vi "main.vi"() -> ()   [LabVIEW 2025]
uses:
  3a10f0c5-8fb2-42eb-acf3-e30270466858.vi
  global/HP amount.vi
  global/bullet amount.vi
  global/difficulty.vi
  global/item amount.vi
  global/demo mode.vi
panel:
  out "Array":bool[](array[boolean])
  out "Player did stuff":bool
  out "Guess bullet type":i32
  out "Numeric":u32
  in  "item array 2":u32[](array[numeric])
  in  "item array":u32[](array[numeric])
  out "item picture 2":u32[](array[ring])
  out "button 2":bool[](array[boolean])
  in  "button":bool[](array[boolean])
  out "item picture":u32[](array[ring])
  out "String":string
  out "chamber ind":u32[](array[ring])
  out "End of action":bool
  out "Total HP var":u32
  out "P1's turn":bool
  out "Chamber":i32[](array[numeric])
  in  "Hit other":bool
  in  "Hit self":bool
  out "STOP":bool
  out "Difficulty":u32
  out "P1 HP var":i32
  out "AI HP var":i32
  out "Item amount":u32
  out "Total rounds":u32
  out "Empty rounds":u32
  out "Live rounds":u32
  out "Player HP ind":T1
  out "AI HP ind":T1
  out "round":u32
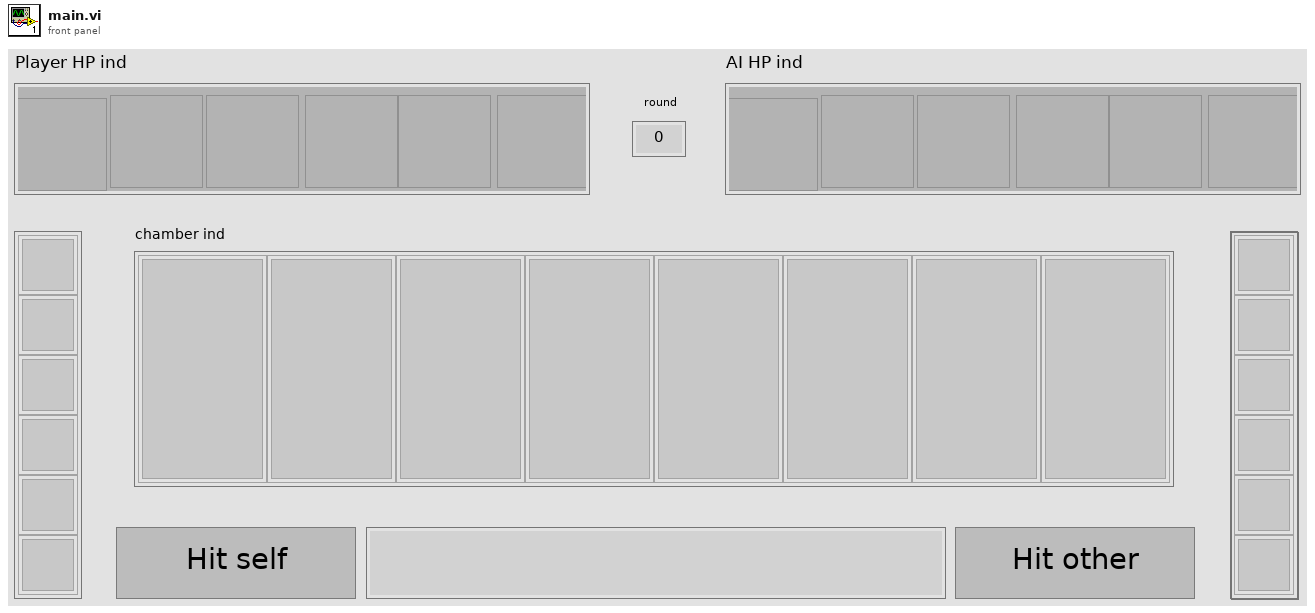
[diagram p1: front panel]
types:
  T1 = cluster{"Boolean":bool, "Boolean 2":bool, "Boolean 3":bool, "Boolean 4":bool, "Boolean 5":bool, "Boolean 6":bool}
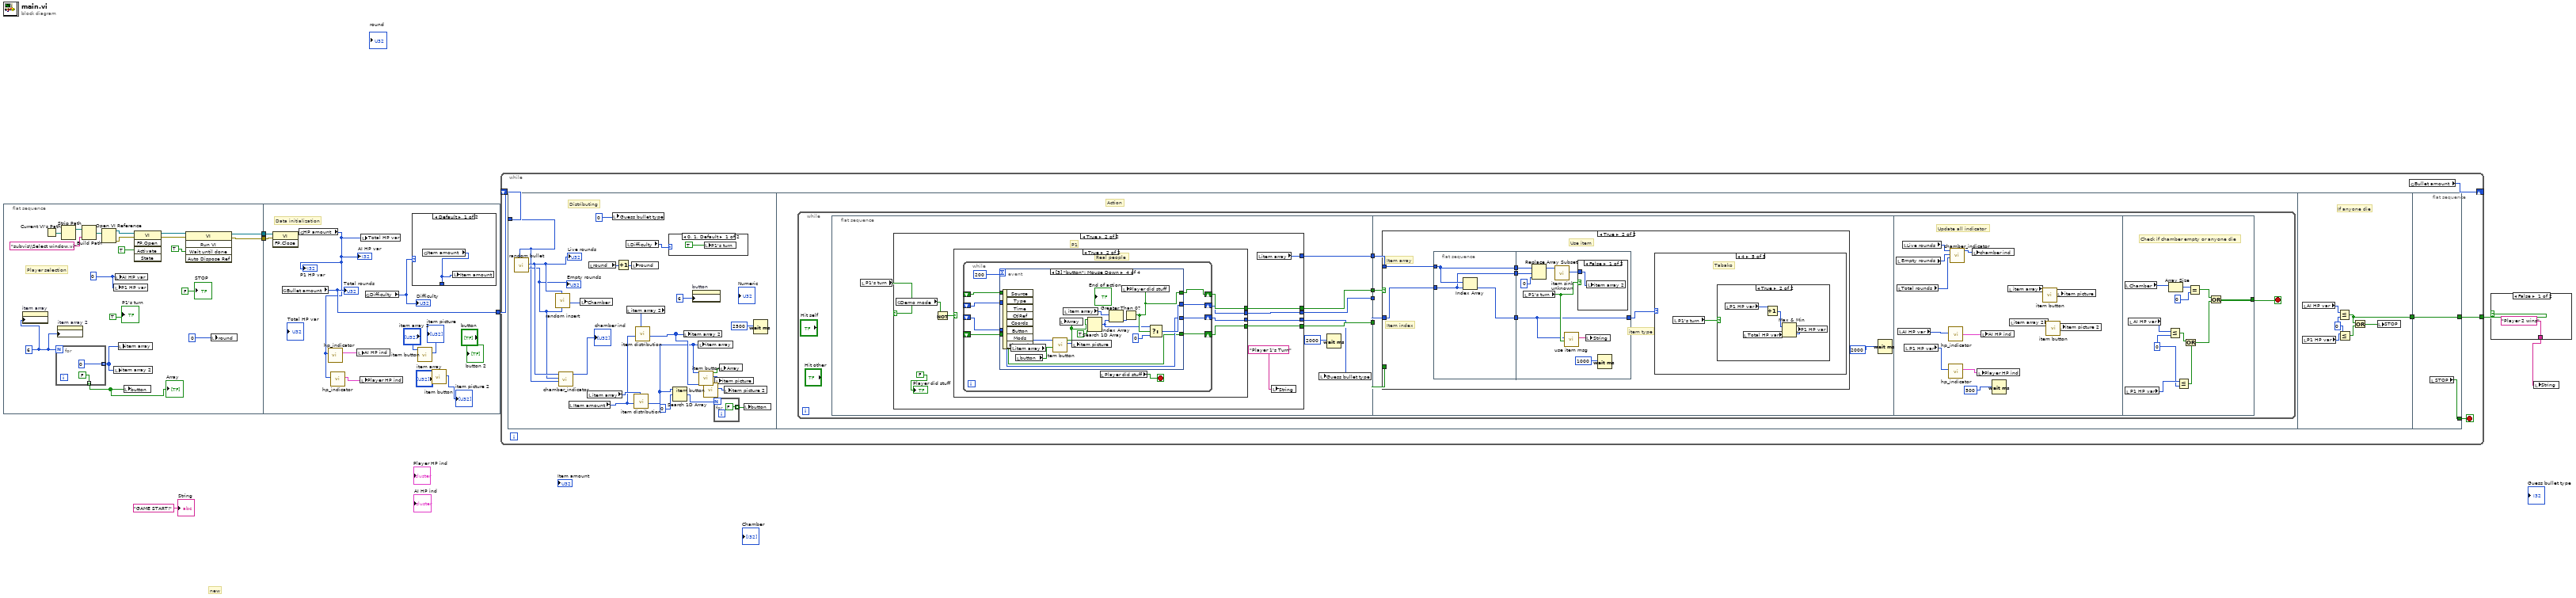
[diagram p0: block diagram]
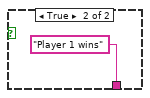
[diagram p2: hidden frame]
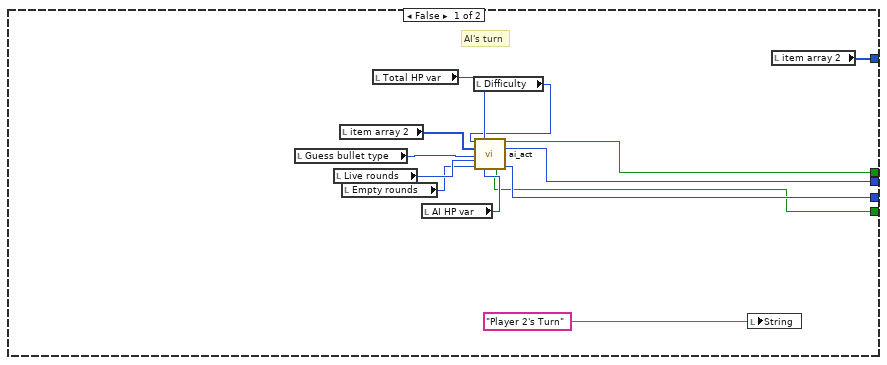
[diagram p4: hidden frame]
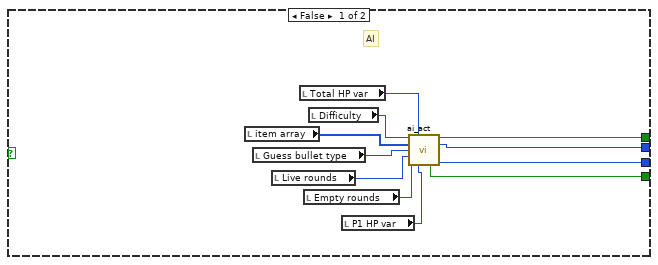
[diagram p5: hidden frame]
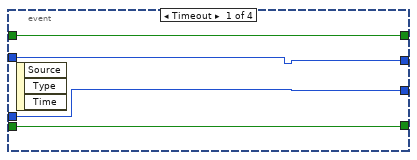
[diagram p6: hidden frame]
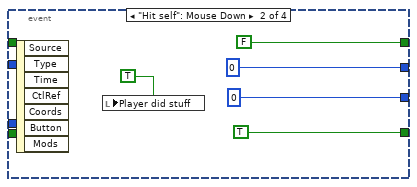
[diagram p7: hidden frame]
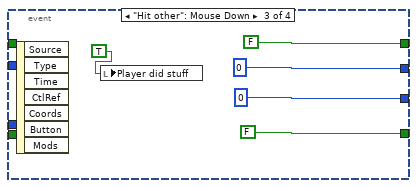
[diagram p8: hidden frame]
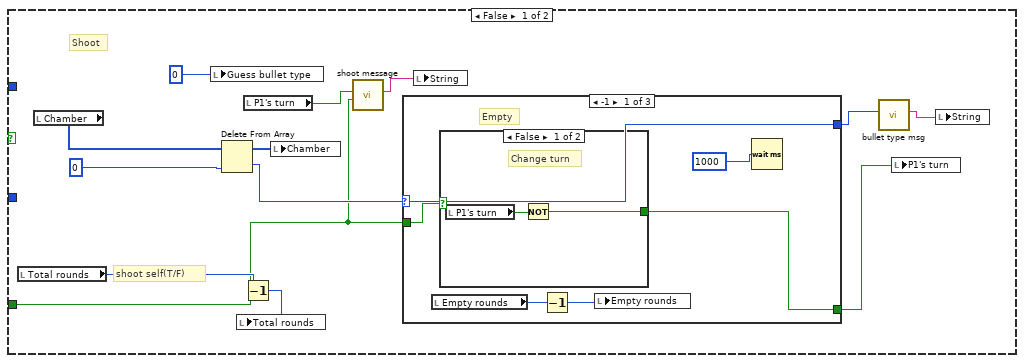
[diagram p9: hidden frame]
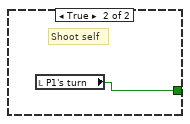
[diagram p10: hidden frame]
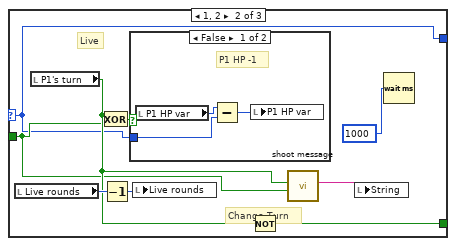
[diagram p11: hidden frame]
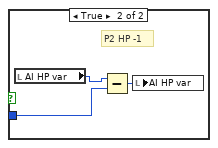
[diagram p12: hidden frame]
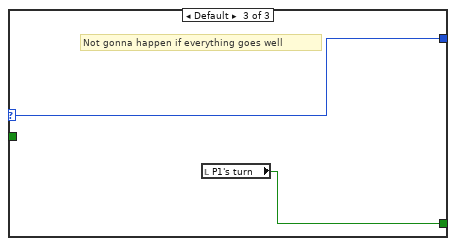
[diagram p13: hidden frame]
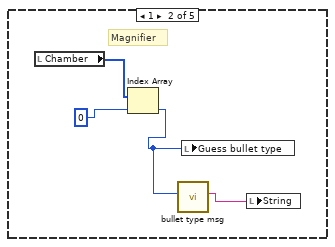
[diagram p15: hidden frame]
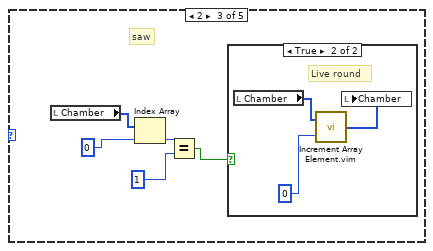
[diagram p16: hidden frame]
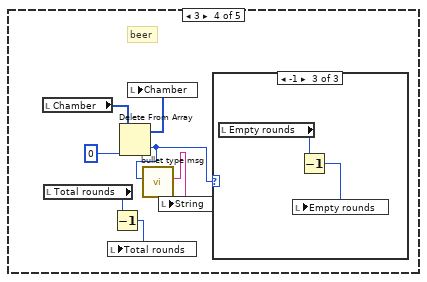
[diagram p18: hidden frame]
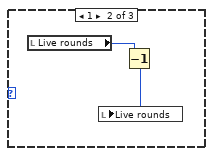
[diagram p20: hidden frame]
diagram:
  # "new"
  n1 = flat-sequence {
    tunnel: [w15] -> w6
    tunnel: [w14] -> w5
    tunnel: w6 -> [w38]
    tunnel: w5 -> [w37]
    tunnel: [w35] -> w1
    frame #0 {
      w9 = u32 6
      w12 = u32 0
      # "Player selection"
      n2 = property on="item array" class="Arr (strict)"("Number of Columns"=w9) -> ()  [unwired: 2 in, 2 out]
      n3 = Current VI's Path() -> (path=w25:path)
      n4 = for {
        N: w9 -> [_]
        tunnel: [u32 0] -> w10 mode=indexing
        tunnel: [FALSE] -> w8 mode=indexing
      }
      "Array" <- w8
      n5 = property on="item array 2" class="Arr (strict)"("Number of Columns"=w9) -> ()  [unwired: 2 in, 2 out]
      n6 = Strip Path(path=w25) -> (stripped path=w24:path)  [unwired: 1 out]
      n7 = Build Path(base path=w24, name or relative path="subvis\\Select window.vi") -> (appended path=w22:path)
      n8 = Open VI Reference(vi path=w22) -> (vi reference=w21:refnum<vi>, error out=w20:errorcluster)  [unwired: 5 in]
      n9 = local write "P1 HP var"(w12) -> ()
      n10 = local write "item array 2"(w10) -> ()
      n11 = local write "AI HP var"(w12) -> ()
      n12 = local write "item array"(w10) -> ()
      n13 = local write "button"(w8) -> ()
      n14 = invoke class="VI" method="FP.Open"(reference=w21, error in=w20, "Activate"=TRUE) -> (reference out=w18:refnum<vi>, error out=w17:errorcluster)  [unwired: 2 in, 3 out]
      n15 = invoke class="VI" method="Run VI"(reference=w18, error in=w17, "Wait until done"=TRUE) -> (reference out=w15:refnum<vi>, error out=w14:errorcluster)  [unwired: 2 in, 3 out]
      n16 = local write "round"(u32 0) -> ()
      "STOP" <- FALSE
      "P1's turn" <- TRUE
    }
    frame #1 {
      # "Data initialization"
      n17 = invoke class="VI" method="FP.Close"(reference=w38, error in=w37) -> ()  [unwired: 1 in, 3 out]
      n18 = global read "bullet amount.vi" "Bullet amount"() -> (w35:u32)
      "Total rounds" <- w35
      n19 = global read "HP amount.vi" "HP amount"() -> (w32:u32)
      "AI HP var" <- w32
      "P1 HP var" <- w32
      n20 = call "hp_indicator.vi"("HP"=w32) -> ("HP pic"=w34:T1)  [unwired: 10 in]
      n21 = call "hp_indicator.vi"("HP"=w32) -> ("HP pic"=w33:T1)  [unwired: 10 in]
      n22 = local write "AI HP ind"(w34) -> ()
      n23 = local write "Player HP ind"(w33) -> ()
      n24 = local write "Total HP var"(w32) -> ()
      n25 = global read "difficulty.vi" "Difficulty"() -> (w36:u32)
      "Difficulty" <- w36
      n26 = case shown="Default" w36 {
        tunnel: [w39 w40] -> _
        frame Default {
          n27 = global read "item amount.vi" "Item amount"() -> (w39:u32)
          n28 = local write "Item amount"(w39) -> ()
        }
        frame 0 {
          w40 = u32 0
          n29 = local write "Item amount"(w40) -> ()
        }
      }
      n30 = call "item button.vi"("item array"="item array 2") -> ("item picture"=→"item picture":u32[])  [unwired: 8 in, 1 out]
      n31 = call "item button.vi"("item array"="item array") -> ("item picture"=→"item picture 2":u32[])  [unwired: 8 in, 1 out]
    }
  }
  n32 = while {
    tunnel: [w45] -> w3
    shift-right: [w42] -> _
    shift-left: w1 -> [w41]
    stop <- w43 stop-if-true
    n33 = flat-sequence {
      tunnel: w41 -> [w61]
      tunnel: [w277] -> w44
      tunnel: [w283] -> w45
      tunnel: w44 -> [w283]
      tunnel: [w282] -> w43
      frame #0 {
        # "Distributing"
        n34 = call "random bullet.vi"("chamber capacity"=w61) -> ("empty rounds"=w64:u32, "live rounds"=w65:u32)  [unwired: 9 in]
        "Live rounds" <- w65
        "Empty rounds" <- w64
        n35 = call "random insert.vi"("empty rounds"=w64, "live rounds"=w65) -> ("chamber"=w67:i32[])  [unwired: 9 in]
        n36 = call "chamber_indicator.vi"("bullet amount"=w61, "empty round"=w64, "live round"=w65) -> ("picture"=→"chamber ind":u32[])  [unwired: 8 in]
        n37 = local read "Item amount"() -> (w59:u32)
        n38 = local write "Chamber"(w67) -> ()
        n39 = local read "item array"() -> (w60:u32[])
        n40 = local read "round"() -> (w47:u32)
        n41 = local write "Guess bullet type"(0) -> ()
        n42 = Increment(x=w47) -> (x+1=w46:u32)
        n43 = local read "Difficulty"() -> (w63:u32)
        n44 = local read "item array 2"() -> (w58:u32[])
        n45 = local write "round"(w46) -> ()
        n46 = call "item distribution.vi"("original items"=w60, "item distributed"=w59) -> ("item"=w50:u32[])  [unwired: 9 in]
        n47 = call "item distribution.vi"("original items"=w58, "item distributed"=w59) -> ("item"=w55:u32[])  [unwired: 9 in]
        n48 = case shown="0, 1, Default" w63 {
          frame 0, 1, Default {
            n49 = local write "P1's turn"(TRUE) -> ()
          }
          frame 2 {
          }
        }
        n50 = Search 1D Array(1D array=w50, element=u32 0) -> (index of element=w48:i32)  [unwired: 1 in]
        n51 = local write "item array 2"(w55) -> ()
        n52 = property on="button" class="Arr"("Number of Rows"=u32 6) -> ()  [unwired: 2 in, 2 out]
        n53 = local write "item array"(w50) -> ()
        n54 = call "item button.vi"("item array"=w50) -> ("confirm"=w54:bool[], "item picture"=w53:u32[])  [unwired: 8 in]
        n55 = call "item button.vi"("item array"=w55) -> ("item picture"=w52:u32[])  [unwired: 8 in, 1 out]
        n56 = for {
          N: w48 -> [_]
          tunnel: [FALSE] -> w51 mode=indexing
        }
        n57 = local write "item picture"(w53) -> ()
        n58 = local write "Array"(w54) -> ()
        n59 = local write "item picture 2"(w52) -> ()
        n60 = local write "button"(w51) -> ()
        n61 = Wait (ms)(milliseconds to wait=u32 2500) -> ()  [unwired: 1 out]
      }
      frame #1 {
        # "Action"
        n62 = while {
          stop <- w71 stop-if-true
          n63 = flat-sequence {
            tunnel: [w79] -> w74
            tunnel: [w78] -> w73
            tunnel: [w77] -> w72
            tunnel: [w76] -> w70
            tunnel: w74 -> [w160]
            tunnel: w73 -> [w157]
            tunnel: w72 -> [w159]
            tunnel: w70 -> [w156]
            tunnel: [w265] -> w71
            frame #0 {
              n64 = local read "P1's turn"() -> (w81:bool)
              n65 = case shown="True" w81 {
                tunnel: [w89 w103] -> w79
                tunnel: [w88 w98] -> w78
                tunnel: [w87 w102] -> w75
                tunnel: [w86 w101] -> w77
                tunnel: [w84 w99] -> w76
                frame False {
                  # "AI's turn"
                  n66 = local read "Guess bullet type"() -> (w83:i32)
                  n67 = local read "Live rounds"() -> (w91:u32)
                  n68 = local read "item array 2"() -> (w82:u32[])
                  n69 = local read "Empty rounds"() -> (w90:u32)
                  n70 = local read "Total HP var"() -> (w94:u32)
                  n71 = local read "AI HP var"() -> (w93:i32)
                  n72 = local read "Difficulty"() -> (w92:u32)
                  n73 = call "ai_act.vi"("difficulty"=w92, "Max health"=w94, "Items"=w82, "current bullet type"=w83, "live rounds"=w91, "empty rounds"=w90, "current health"=w93) -> ("use item"=w89:bool, "item index"=w88:i32, "shoot self"=w86:bool, "Guess type"=w87:i32)  [unwired: 5 in]
                  n74 = local write "String"("Player 2's Turn") -> ()
                  n75 = local read "item array 2"() -> (w84:u32[])
                }
                frame True {
                  # "P1"
                  n76 = global read "demo mode.vi" "Demo mode"() -> (w95:bool)
                  n77 = Not(x=w95) -> (.not. x?=w96:bool)
                  n78 = case shown="True" w96 {
                    tunnel: [w109 w118] -> w103
                    tunnel: [w108 w117] -> w98
                    tunnel: [w107 w116] -> w102
                    tunnel: [w106 w115] -> w101
                    frame False {
                      # "AI"
                      n79 = local read "item array"() -> (w104:u32[])
                      n80 = local read "Guess bullet type"() -> (w105:i32)
                      n81 = local read "Live rounds"() -> (w112:u32)
                      n82 = local read "Total HP var"() -> (w114:u32)
                      n83 = local read "Empty rounds"() -> (w111:u32)
                      n84 = local read "Difficulty"() -> (w113:u32)
                      n85 = local read "P1 HP var"() -> (w110:i32)
                      n86 = call "ai_act.vi"("difficulty"=w113, "Max health"=w114, "Items"=w104, "current bullet type"=w105, "live rounds"=w112, "empty rounds"=w111, "current health"=w110) -> ("use item"=w109:bool, "item index"=w108:i32, "shoot self"=w106:bool, "Guess type"=w107:i32)  [unwired: 5 in]
                    }
                    frame True {
                      # "Real people"
                      n87 = while {
                        shift-right: [w126] -> w118
                        shift-left: _ -> [w122]
                        shift-right: [w125] -> w117
                        shift-left: _ -> [w121]
                        shift-right: [w124] -> w116
                        shift-left: _ -> [w120]
                        shift-right: [w123] -> w115
                        shift-left: _ -> [w119]
                        stop <- w128 stop-if-true
                        n88 = event shown="[3] \"button\": Mouse Down" {
                          selector: _ -> [_ _ _ _]
                          dyn-events: _ -> [_ _ _ _]
                          timeout: 200 -> [_ _ _ _]
                          tunnel: [w132 FALSE FALSE w148] -> w126
                          tunnel: [w131 u32 0 u32 0 w146] -> w125
                          tunnel: [w130 0 0 w145] -> w124
                          tunnel: [w129 TRUE FALSE w144] -> w123
                          tunnel: w122 -> [w132 _ _ _]
                          tunnel: w121 -> [w131 _ _ _]
                          tunnel: w120 -> [w130 _ _ w145]
                          tunnel: w119 -> [w129 _ _ w144]
                          event Timeout {
                            n89 = event-data() -> ()  [unwired: 1 in, 3 out]
                          }
                          event "Hit self": Mouse Down {
                            n90 = event-data() -> ()  [unwired: 1 in, 7 out]
                            n91 = local write "Player did stuff"(TRUE) -> ()
                          }
                          event "Hit other": Mouse Down {
                            n92 = event-data() -> ()  [unwired: 1 in, 7 out]
                            n93 = local write "Player did stuff"(TRUE) -> ()
                          }
                          event "button": Mouse Down {
                            n94 = event-data() -> ()  [unwired: 1 in, 8 out]
                            n95 = local read "item array"() -> (w155:u32[])
                            n96 = local read "button"() -> (w154:bool[])
                            n97 = call "item button.vi"("item array"=w155, "button"=w154) -> ("confirm"=w152:bool[], "item picture"=w153:u32[])  [unwired: 7 in]
                            n98 = local write "Array"(w152) -> ()
                            n99 = local read "item array"() -> (w150:u32[])
                            n100 = local write "item picture"(w153) -> ()
                            n101 = Search 1D Array(1D array=w152, element=TRUE) -> (index of element=w147:i32)  [unwired: 1 in]
                            n102 = Index Array(array=w150, index=w147) -> (element=w149:u32)
                            n103 = Greater Than 0?(x=w149) -> (x > 0?=w148:bool)
                            n104 = local write "Player did stuff"(w148) -> ()
                            n105 = Select(t=w147, s=w148, f=0) -> (s? t:f=w146:i32)
                          }
                        }
                        n106 = local read "Player did stuff"() -> (w128:bool)
                      }
                    }
                  }
                  n107 = local read "item array"() -> (w99:u32[])
                  n108 = local write "String"("Player 1's Turn") -> ()
                  "Player did stuff" <- FALSE
                }
              }
              n109 = local write "Guess bullet type"(w75) -> ()
              n110 = Wait (ms)(milliseconds to wait=u32 2000) -> ()  [unwired: 1 out]
            }
            frame #1 {
              n111 = case shown="True" w160 {
                tunnel: w159 -> [w163 _]
                tunnel: w157 -> [_ w201]
                tunnel: w156 -> [_ w205]
                frame False {
                  # "shoot self(T/F)"
                  # "Shoot"
                  n112 = local read "Total rounds"() -> (w169:u32)
                  n113 = local read "Chamber"() -> (w173:i32[])
                  n114 = local write "Guess bullet type"(0) -> ()
                  n115 = Delete From Array(array=w173, index=0) -> (deleted portion=w171:i32, array with subset deleted=w170:i32[])  [unwired: 1 in]
                  n116 = Decrement(x=w169) -> (x-1=w168:u32)
                  n117 = local write "Total rounds"(w168) -> ()
                  n118 = local read "P1's turn"() -> (w162:bool)
                  n119 = local write "Chamber"(w170) -> ()
                  n120 = call "shoot message.vi"("shoot self"=w163, "P1 Turn"=w162) -> ("String"=w161:string)  [unwired: 9 in]
                  n121 = case shown="-1" w171 {
                    selector: w171 -> [w175 w183 w198]
                    tunnel: w163 -> [w176 w185 _]
                    tunnel: [w177 w188 w199] -> w167
                    tunnel: [w175 w183 w198] -> w165
                    frame -1 {
                      # "Empty"
                      n122 = local read "Empty rounds"() -> (w179:u32)
                      n123 = case shown="False" w176 {
                        tunnel: [w180 w182] -> w177
                        frame False {
                          # "Change turn"
                          n124 = local read "P1's turn"() -> (w181:bool)
                          n125 = Not(x=w181) -> (.not. x?=w180:bool)
                        }
                        frame True {
                          # "Shoot self"
                          n126 = local read "P1's turn"() -> (w182:bool)
                        }
                      }
                      n127 = Decrement(x=w179) -> (x-1=w178:u32)
                      n128 = local write "Empty rounds"(w178) -> ()
                      n129 = Wait (ms)(milliseconds to wait=u32 1000) -> ()  [unwired: 1 out]
                    }
                    frame 1, 2 {
                      # "Change Turn"
                      # "Live"
                      n130 = local read "Live rounds"() -> (w190:u32)
                      n131 = local read "P1's turn"() -> (w186:bool)
                      n132 = Exclusive Or(1:w185, 2:w186) -> (0:w191:bool)
                      n133 = Decrement(x=w190) -> (x-1=w189:u32)
                      n134 = case shown="False" w191 {
                        tunnel: w183 -> [w192 w195]
                        frame False {
                          # "P1 HP -1"
                          n135 = local read "P1 HP var"() -> (w193:i32)
                          n136 = Subtract(x=w193, y=w192) -> (x-y=w194:i32)
                          n137 = local write "P1 HP var"(w194) -> ()
                        }
                        frame True {
                          # "P2 HP -1"
                          n138 = local read "AI HP var"() -> (w196:i32)
                          n139 = Subtract(x=w196, y=w195) -> (x-y=w197:i32)
                          n140 = local write "AI HP var"(w197) -> ()
                        }
                      }
                      n141 = local write "Live rounds"(w189) -> ()
                      n142 = Not(x=w186) -> (.not. x?=w188:bool)
                      n143 = call "shoot message.vi"("shoot self"=w185, "P1 Turn"=w186) -> ("String"=w187:string)  [unwired: 9 in]
                      n144 = local write "String"(w187) -> ()
                      n145 = Wait (ms)(milliseconds to wait=u32 1000) -> ()  [unwired: 1 out]
                    }
                    frame Default {
                      # "Not gonna happen if everything goes well"
                      n146 = local read "P1's turn"() -> (w199:bool)
                    }
                  }
                  n147 = local write "String"(w161) -> ()
                  n148 = call "bullet type msg.vi"("bullet type"=w165) -> ("String"=w164:string)  [unwired: 10 in]
                  n149 = local write "P1's turn"(w167) -> ()
                  n150 = local write "String"(w164) -> ()
                }
                frame True {
                  # "item type"
                  # "Item array"
                  # "Item index"
                  # "Use item"
                  n151 = flat-sequence {
                    tunnel: w205 -> [w240]
                    tunnel: [w239] -> w204
                    tunnel: [w240] -> w203
                    tunnel: w201 -> [w238]
                    tunnel: [w238] -> w200
                    tunnel: w204 -> [w244]
                    tunnel: w203 -> [w249]
                    tunnel: [w244] -> w202
                    tunnel: w200 -> [w241]
                    frame #0 {
                      n152 = Index Array(array=w240, index=w238) -> (element=w239:u32)
                    }
                    frame #1 {
                      n153 = local read "P1's turn"() -> (w245:bool)
                      n154 = Replace Array Subset(array=w249, new element=u32 0, index=w241) -> (w247:u32[])
                      n155 = call "item sink unknown.vi"("Items in"=w247) -> ("Items out"=w246:u32[])  [unwired: 10 in]
                      n156 = call "use item msg.vi"("P1 turn"=w245, "Item num"=w244) -> ("String"=w243:string)  [unwired: 9 in]
                      n157 = case shown="False" w245 {
                        tunnel: w246 -> [w250 w251]
                        frame False {
                          n158 = local write "item array 2"(w250) -> ()
                        }
                        frame True {
                          n159 = local write "item array"(w251) -> ()
                        }
                      }
                      n160 = local write "String"(w243) -> ()
                      n161 = Wait (ms)(milliseconds to wait=u32 1000) -> ()  [unwired: 1 out]
                    }
                  }
                  n162 = case shown="4" w202 {
                    frame 0, Default {
                      # "Should not happen"
                    }
                    frame 1 {
                      # "Magnifier"
                      n163 = local read "Chamber"() -> (w209:i32[])
                      n164 = Index Array(array=w209, index=0) -> (element=w207:i32)
                      n165 = call "bullet type msg.vi"("bullet type"=w207) -> ("String"=w206:string)  [unwired: 10 in]
                      n166 = local write "Guess bullet type"(w207) -> ()
                      n167 = local write "String"(w206) -> ()
                    }
                    frame 2 {
                      # "saw"
                      n168 = local read "Chamber"() -> (w213:i32[])
                      n169 = Index Array(array=w213, index=0) -> (element=w212:i32)
                      n170 = Equal?(x=w212, y=1) -> (x = y?=w210:bool)
                      n171 = case shown="True" w210 {
                        frame False {
                          # "Empty round"
                        }
                        frame True {
                          # "Live round"
                          n172 = local read "Chamber"() -> (w216:i32[])
                          n173 = call "Increment Array Element.vim"("index"=0, "array in"=w216) -> ("array out"=w217:i32[])
                          n174 = local write "Chamber"(w217) -> ()
                        }
                      }
                    }
                    frame 3 {
                      # "beer"
                      n175 = local read "Chamber"() -> (w223:i32[])
                      n176 = local read "Total rounds"() -> (w220:u32)
                      n177 = Decrement(x=w220) -> (x-1=w221:u32)
                      n178 = local write "Total rounds"(w221) -> ()
                      n179 = Delete From Array(array=w223, index=0) -> (deleted portion=w219:i32, array with subset deleted=w222:i32[])  [unwired: 1 in]
                      n180 = local write "Chamber"(w222) -> ()
                      n181 = call "bullet type msg.vi"("bullet type"=w219) -> ("String"=w218:string)  [unwired: 10 in]
                      n182 = local write "String"(w218) -> ()
                      n183 = case shown="-1" w219 {
                        frame 0, Default {
                        }
                        frame 1 {
                          n184 = local read "Live rounds"() -> (w226:u32)
                          n185 = Decrement(x=w226) -> (x-1=w225:u32)
                          n186 = local write "Live rounds"(w225) -> ()
                        }
                        frame -1 {
                          n187 = local read "Empty rounds"() -> (w228:u32)
                          n188 = Decrement(x=w228) -> (x-1=w227:u32)
                          n189 = local write "Empty rounds"(w227) -> ()
                        }
                      }
                    }
                    frame 4 {
                      # "Tabako"
                      n190 = local read "P1's turn"() -> (w229:bool)
                      n191 = case shown="True" w229 {
                        frame False {
                          n192 = local read "AI HP var"() -> (w233:i32)
                          n193 = local read "Total HP var"() -> (w231:u32)
                          n194 = Increment(x=w233) -> (x+1=w232:i32)
                          n195 = Max & Min(x=w232, y=w231) -> (min(x,y)=w230:u32)  [unwired: 1 out]
                          n196 = local write "AI HP var"(w230) -> ()
                        }
                        frame True {
                          n197 = local read "P1 HP var"() -> (w237:i32)
                          n198 = local read "Total HP var"() -> (w235:u32)
                          n199 = Increment(x=w237) -> (x+1=w236:i32)
                          n200 = Max & Min(x=w236, y=w235) -> (min(x,y)=w234:u32)  [unwired: 1 out]
                          n201 = local write "P1 HP var"(w234) -> ()
                        }
                      }
                    }
                  }
                }
              }
              n202 = Wait (ms)(milliseconds to wait=u32 2000) -> ()  [unwired: 1 out]
            }
            frame #2 {
              # "Update all indicator"
              n203 = local read "Empty rounds"() -> (w262:u32)
              n204 = local read "Total rounds"() -> (w261:u32)
              n205 = local read "AI HP var"() -> (w259:i32)
              n206 = local read "Live rounds"() -> (w263:u32)
              n207 = local read "P1 HP var"() -> (w258:i32)
              n208 = call "hp_indicator.vi"("HP"=w259) -> ("HP pic"=w257:T1)  [unwired: 10 in]
              n209 = call "hp_indicator.vi"("HP"=w258) -> ("HP pic"=w256:T1)  [unwired: 10 in]
              n210 = call "chamber_indicator.vi"("bullet amount"=w261, "empty round"=w262, "live round"=w263) -> ("picture"=w264:u32[])  [unwired: 8 in]
              n211 = local write "chamber ind"(w264) -> ()
              n212 = local write "Player HP ind"(w256) -> ()
              n213 = local write "AI HP ind"(w257) -> ()
              n214 = Wait (ms)(milliseconds to wait=u32 500) -> ()  [unwired: 1 out]
              n215 = local read "item array"() -> (w255:u32[])
              n216 = local read "item array 2"() -> (w253:u32[])
              n217 = call "item button.vi"("item array"=w255) -> ("item picture"=w254:u32[])  [unwired: 8 in, 1 out]
              n218 = call "item button.vi"("item array"=w253) -> ("item picture"=w252:u32[])  [unwired: 8 in, 1 out]
              n219 = local write "item picture"(w254) -> ()
              n220 = local write "item picture 2"(w252) -> ()
            }
            frame #3 {
              w266 = 0
              # "Check if chamber empty or anyone die"
              n221 = local read "Chamber"() -> (w273:i32[])
              n222 = local read "P1 HP var"() -> (w271:i32)
              n223 = local read "AI HP var"() -> (w272:i32)
              n224 = Less Or Equal?(x=w272, y=w266) -> (x <= y?=w269:bool)
              n225 = Array Size(array=w273) -> (size(s)=w275:i32)
              n226 = Less Or Equal?(x=w271, y=w266) -> (x <= y?=w268:bool)
              n227 = Or(x=w269, y=w268) -> (x .or. y?=w267:bool)
              n228 = Equal?(x=w275, y=0) -> (x = y?=w270:bool)
              n229 = Or(x=w270, y=w267) -> (x .or. y?=w265:bool)
            }
          }
        }
      }
      frame #2 {
        w281 = 0
        # "If anyone die"
        n230 = local read "AI HP var"() -> (w278:i32)
        n231 = local read "P1 HP var"() -> (w279:i32)
        n232 = Less Or Equal?(x=w278, y=w281) -> (x <= y?=w277:bool)
        n233 = Less Or Equal?(x=w279, y=w281) -> (x <= y?=w280:bool)
        n234 = Or(x=w277, y=w280) -> (x .or. y?=w276:bool)
        n235 = local write "STOP"(w276) -> ()
      }
      frame #3 {
        n236 = local read "STOP"() -> (w282:bool)
      }
    }
    n237 = global read "bullet amount.vi" "Bullet amount"() -> (w42:u32)
  }
  n238 = case shown="False" w3 {
    tunnel: ["Player 2 wins" "Player 1 wins"] -> w2
    frame False {
    }
    frame True {
    }
  }
  n239 = local write "String"(w2) -> ()
  "String" <- "GAME START!" ("String")
